vi "AlliGator Save FLI Dataset Metadata to HDF5.vi"(7 "Compression":bool, 8 "error in (no error)":errorcluster, 9 "Gate Names":string[](array[string])=["Gate"], 10 "Dataset Information":T1, 11 "Software + Version":string) -> (0 "error out":errorcluster, 2 "File Path out":path, 3 "HDF5 File ref out":T3 format="%.0x")   [LabVIEW 2021, in "AlliGator Files.lvlib"]
doc: "Saves the FLI Dataset metadata in the AlliGator HDF5 file format."
uses:
  AlliGator Files.lvlib
  <vilib>/addons/h5labview2/base/hid_t.ctl
  AlliGator Saved Dataset Information.ctl
  Phasor/Phasor Fluorescence Lifetime Parameters v3.ctl
  <vilib>/addons/h5labview2/file/H5Fmode.ctl
  AlliGator FLI Dataset HDF5 File Sections.ctl
  Source Image/AlliGator Image Binning Options.ctl
  <vilib>/addons/h5labview2/base/lib_path.vi
  <vilib>/addons/h5labview2/base/H5Equery.vi
  <vilib>/addons/h5labview2/dataset/H5Dwrite.llb/H5Dwrite.xnode
  <vilib>/addons/h5labview2/group/H5G.lvlib
  Strings/Strings.lvlib
  Utilities/Utilities.lvlib
  Source Image/AlliGator Source Image.lvlib
  <vilib>/addons/h5labview2/file/H5F.lvlib
  Phasor/Phasor.lvlib
panel:
  # "see the AlliGator License on the block diagram (Ctrl+E or Window:Show Block Diagram)"
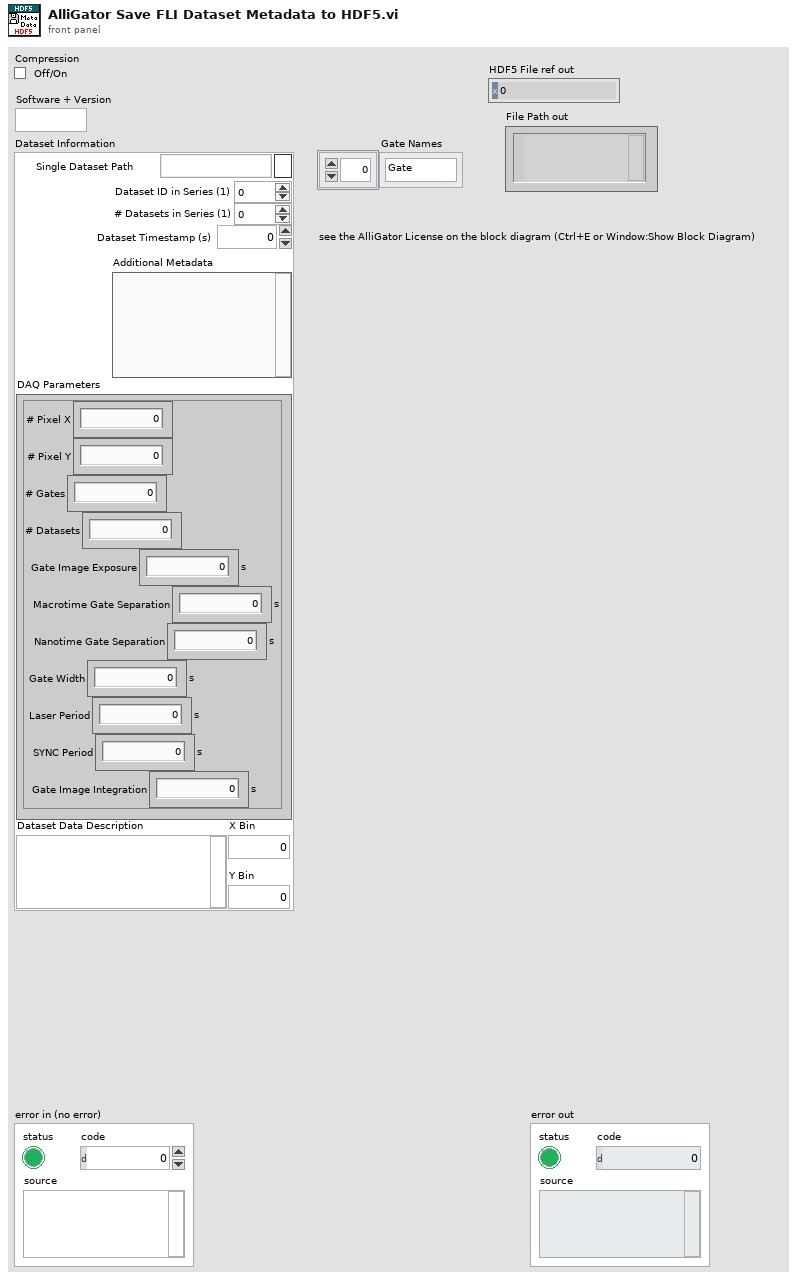
[diagram p1: front panel]
types:
  T1 = typedef "AlliGator Files.lvlib/AlliGator Saved Dataset Information.ctl" = cluster{"Single Dataset Path":path, "Dataset ID in Series (1)":i32, "# Datasets in Series (1)":i32, "Dataset Timestamp (s)":dbl, "Additional Metadata":string, "DAQ Parameters":T2, "Dataset Data Description":string, "X Bin":i32, "Y Bin":i32}
  T2 = typedef "Phasor.lvlib/Phasor Fluorescence Lifetime Parameters v3.ctl" = cluster{"# Pixel X":i32, "# Pixel Y":i32, "# Gates":i32, "# Datasets":i32, "Gate Image Exposure":dbl[unit], "Macrotime Gate Separation":dbl[unit], "Nanotime Gate Separation":dbl[unit], "Gate Width":dbl[unit], "Laser Period":dbl[unit], "SYNC Period":dbl[unit], "Gate Image Integration":dbl[unit]}
  T3 = typedef "hid_t.ctl" = i64
  T4 = typedef "AlliGator Files.lvlib/AlliGator FLI Dataset HDF5 File Sections.ctl" = enum16{"File Information", "DAQ Parameters", "Image Information", "Metadata"}
  T5 = typedef "H5F.lvlib/H5Fmode.ctl" = enum16{"read-only", "read-write", "overwrite", "create new", "open or create"}
  T6 = typedef "AlliGator Source Image.lvlib/AlliGator Image Binning Options.ctl" = cluster{"Use Image Binning":bool, "X Bin":i32, "Y Bin":i32}
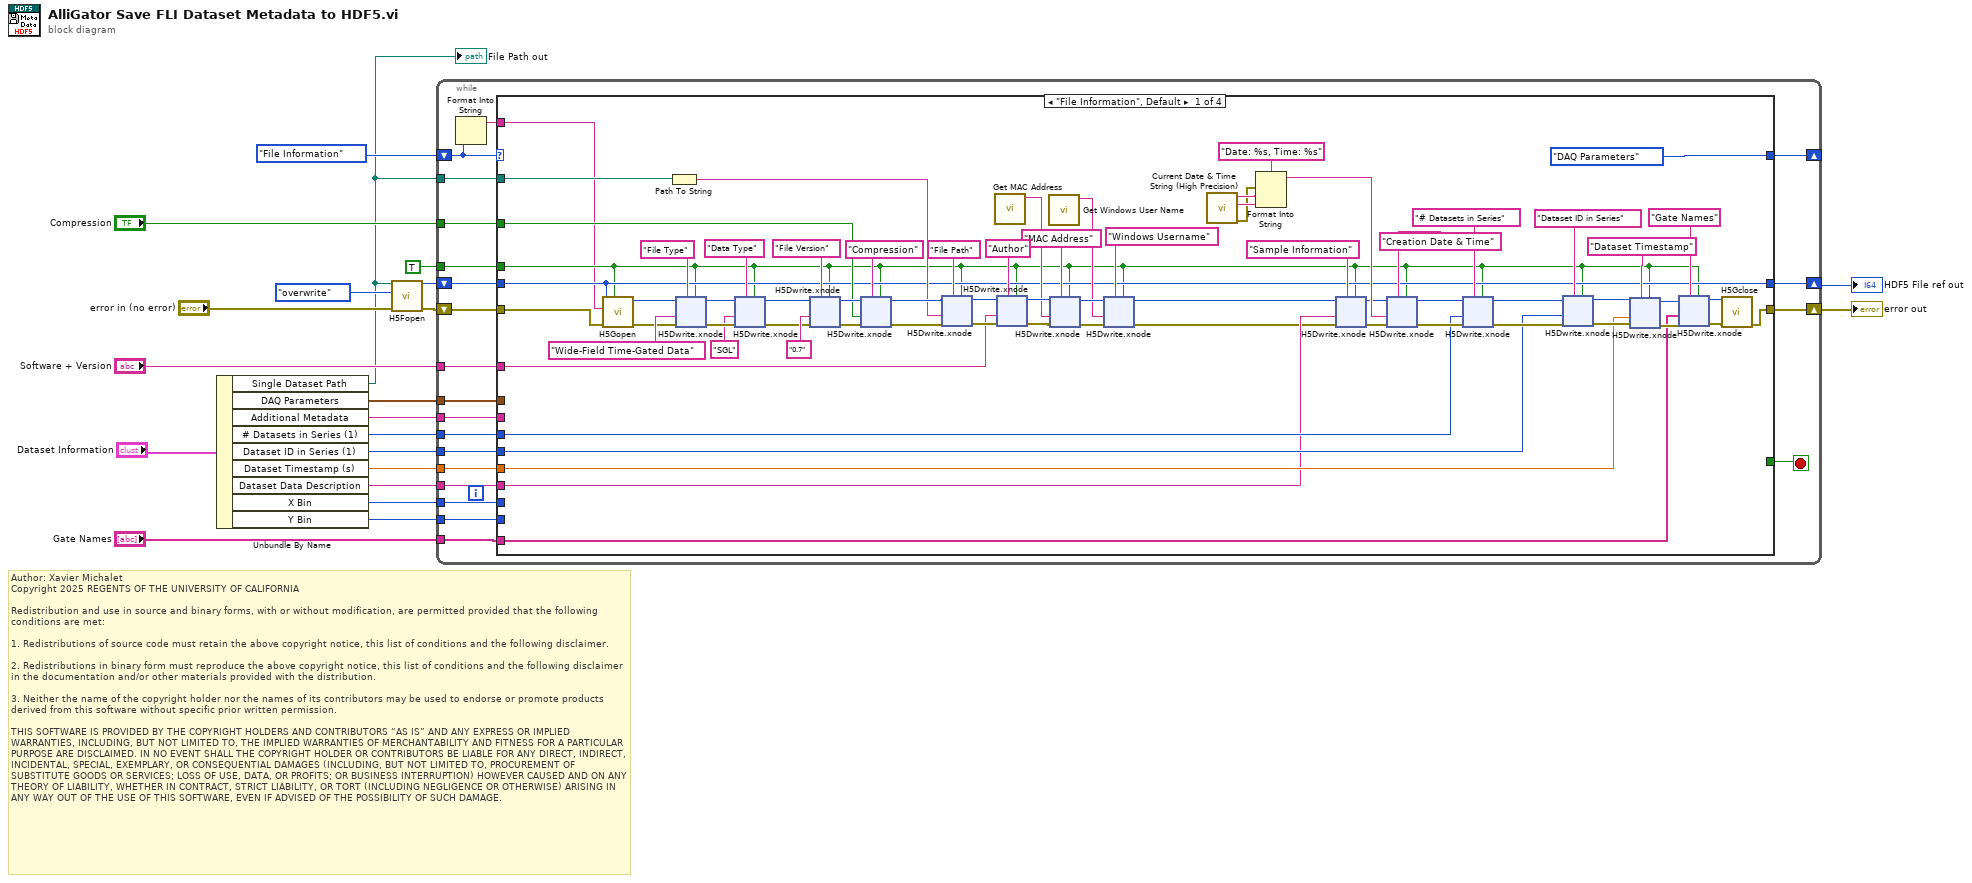
[diagram p0: block diagram]
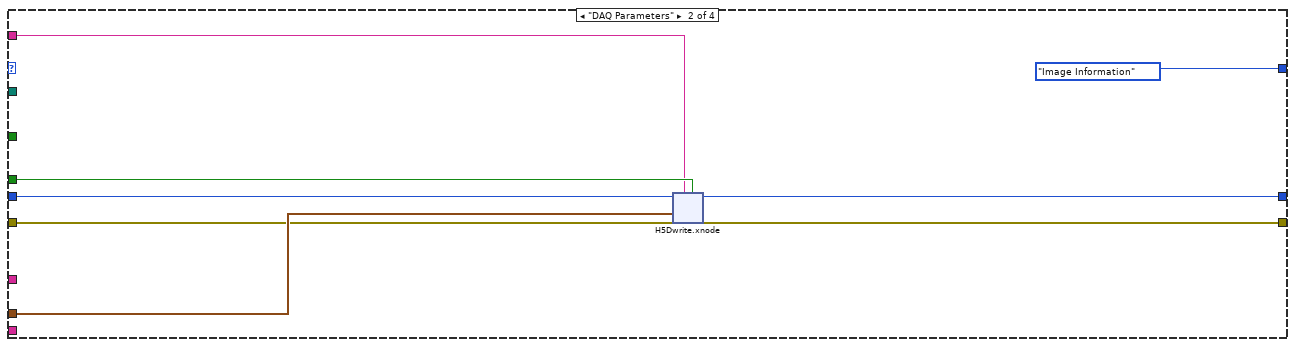
[diagram p2: hidden frame]
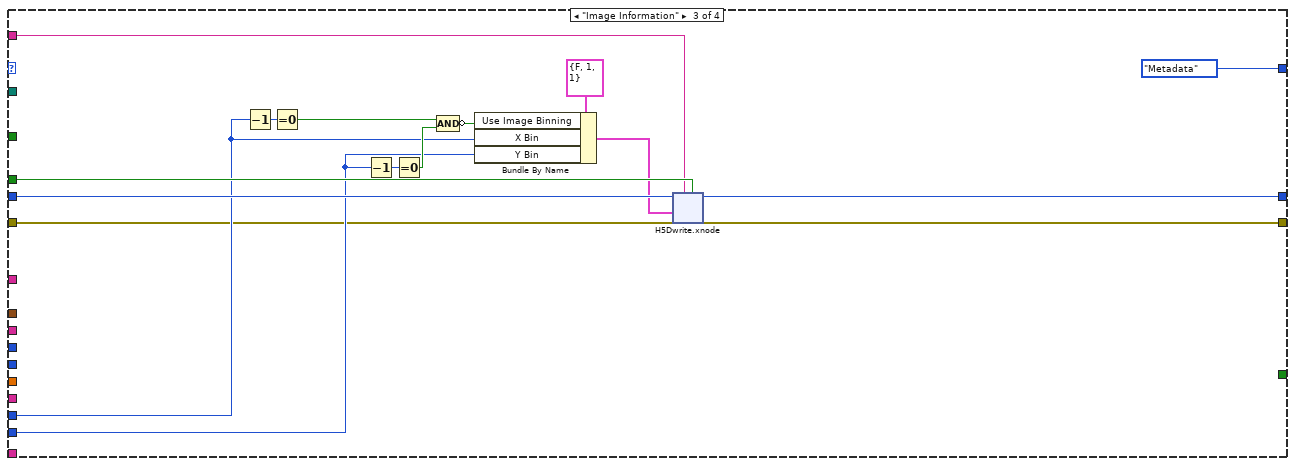
[diagram p3: hidden frame]
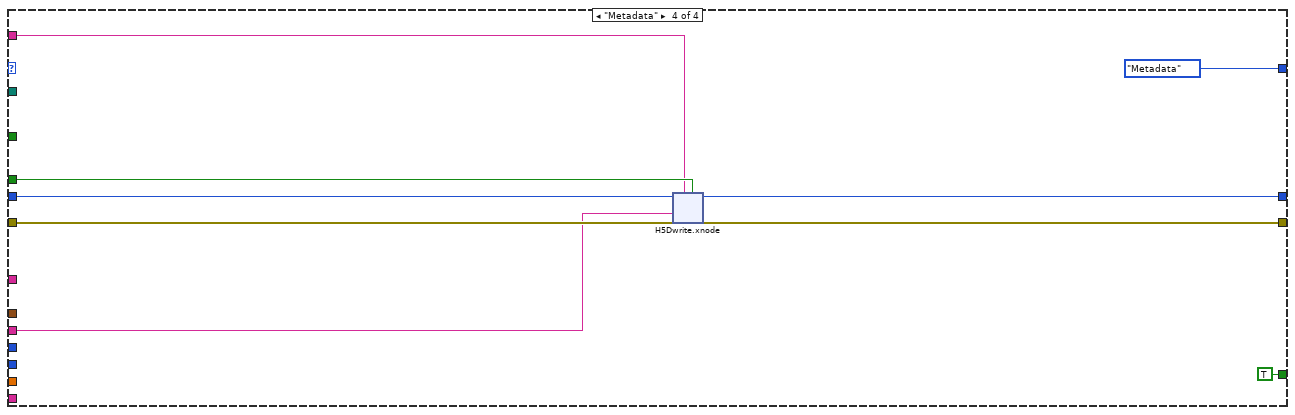
[diagram p4: hidden frame]
diagram:
  # "Author: Xavier Michalet\nCopyright 2025 REGENTS OF THE UNIVERSITY OF CALIFORNIA\n\nRedistribution and use in source and binary forms, with or without modification, are permitted provided that the following conditions are met:\n\n1. Redistributions of source code must retain the above copyright notice, this list of conditions and the following disclaimer.\n\n2. Redistributions in binary form must reproduce the above copyright notice, this list of conditions and the following disclaimer in the documentation and/or other materials provided with the distribution.\n\n3. Neither the name of the copyright holder nor the names of its contributors may be used to endorse or promote products derived from this software without specific prior written permission.\n\nTHIS SOFTWARE IS PROVIDED BY THE COPYRIGHT HOLDERS AND CONTRIBUTORS “AS IS” AND ANY EXPRESS OR IMPLIED WARRANTIES, INCLUDING, BUT NOT LIMITED TO, THE IMPLIED WARRANTIES OF MERCHANTABILITY AND FITNESS FOR A PARTICULAR PURPOSE ARE DISCLAIMED. IN NO EVENT SHALL THE COPYRIGHT HOLDER OR CONTRIBUTORS BE LIABLE FOR ANY DIRECT, INDIRECT, INCIDENTAL, SPECIAL, EXEMPLARY, OR CONSEQUENTIAL DAMAGES (INCLUDING, BUT NOT LIMITED TO, PROCUREMENT OF SUBSTITUTE GOODS OR SERVICES; LOSS OF USE, DATA, OR PROFITS; OR BUSINESS INTERRUPTION) HOWEVER CAUSED AND ON ANY THEORY OF LIABILITY, WHETHER IN CONTRACT, STRICT LIABILITY, OR TORT (INCLUDING NEGLIGENCE OR OTHERWISE) ARISING IN ANY WAY OUT OF THE USE OF THIS SOFTWARE, EVEN IF ADVISED OF THE POSSIBILITY OF SUCH DAMAGE."
  n1 = Unbundle By Name("Dataset Information") -> ("Single Dataset Path"=w1:path, "DAQ Parameters"=w13:T2, "Additional Metadata"=w15:string, "# Datasets in Series (1)"=w8:i32, "Dataset ID in Series (1)"=w9:i32, "Dataset Timestamp (s)"=w10:dbl, "Dataset Data Description"=w16:string, "X Bin"=w17:i32, "Y Bin"=w18:i32)
  "File Path out" <- w1
  n2 = call <vilib>:"H5Fopen.vi"("error in (no error)"="error in (no error)", "mode (read-only)"=H5Fmode."overwrite", "path"=w1) -> ("error out"=w3:errorcluster, "ref out"=w14:T3)  [unwired: 7 in]
  n3 = while {
    tunnel: "Compression" -> [w39]
    tunnel: "Software + Version" -> [w38]
    tunnel: w8 -> [w37]
    tunnel: w9 -> [w36]
    tunnel: w10 -> [w35]
    tunnel: w1 -> [w34]
    tunnel: "Gate Names" -> [w33]
    shift-right: [w40] -> w21
    shift-left: w3 -> [w42]
    tunnel: TRUE ("replace? (F)") -> [w32]
    shift-right: [w31] -> _
    shift-left: AlliGator_FLI_Dataset_HDF5_File_Sections."File Information" -> [w28]
    shift-right: [w30] -> w19
    shift-left: w14 -> [w41]
    tunnel: w13 -> [w29]
    tunnel: w15 -> [w26]
    tunnel: w16 -> [w24]
    tunnel: w17 -> [w23]
    tunnel: w18 -> [w22]
    stop <- w25 stop-if-true
    n4 = Format Into String(w28) -> (resulting string=w27:string)  [unwired: 3 in, 1 out]
    n5 = case shown="\"File Information\", Default" w28 {
      tunnel: w42 -> [w111 w383 w405 w447]
      tunnel: w41 -> [w48 w384 w420 w448]
      tunnel: [w104 w381 w418 w445] -> w40
      tunnel: w39 -> [w95 _ _ _]
      tunnel: w38 -> [w62 _ _ _]
      tunnel: w37 -> [w58 _ _ _]
      tunnel: w36 -> [w57 _ _ _]
      tunnel: w35 -> [w56 _ _ _]
      tunnel: w34 -> [w50 _ _ _]
      tunnel: w33 -> [w49 _ _ _]
      tunnel: w32 -> [w47 w380 w417 w444]
      tunnel: [AlliGator_FLI_Dataset_HDF5_File_Sections."DAQ Parameters" AlliGator_FLI_Dataset_HDF5_File_Sections."Image Information" AlliGator_FLI_Dataset_HDF5_File_Sections."Metadata" AlliGator_FLI_Dataset_HDF5_File_Sections."Metadata"] -> w31
      tunnel: [w48 w382 w419 w446] -> w30
      tunnel: w29 -> [_ w385 _ _]
      tunnel: w27 -> [w46 w379 w416 w443]
      tunnel: w26 -> [_ _ _ w442]
      tunnel: [_ _ _ TRUE] -> w25
      tunnel: w24 -> [w44 _ _ _]
      tunnel: w23 -> [_ _ w407 _]
      tunnel: w22 -> [_ _ w406 _]
      frame "File Information", Default {
        n6 = call <vilib>:"H5Gopen.vi"("create? (F)"=w47, "error in (no error)"=w111, "name"=w46, "ref in"=w48) -> ("error out"=w108:errorcluster, "group out"=w106:T3)  [unwired: 6 in]
        n7 = Path To String(path=w50) -> (string=w79:string)
        n8 = xnode "H5Dwrite.xnode"("replace? (F)"=w47, "dataset name"="File Type", "error in (no error)"=w108, "data"="Wide-Field Time-Gated Data" ("dataset name"), "ref in"=w106) -> ("error out"=w102:errorcluster, "ref out"=w103:T3)  [unwired: 2 in, 1 out]
        n9 = xnode "H5Dwrite.xnode"("replace? (F)"=w47, "dataset name"="Data Type", "error in (no error)"=w102, "data"="SGL" ("dataset name"), "ref in"=w103) -> ("error out"=w100:errorcluster, "ref out"=w101:T3)  [unwired: 2 in, 1 out]
        n10 = xnode "H5Dwrite.xnode"("replace? (F)"=w47, "dataset name"="File Version", "error in (no error)"=w100, "data"="0.7" ("dataset name"), "ref in"=w101) -> ("error out"=w96:errorcluster, "ref out"=w97:T3)  [unwired: 2 in, 1 out]
        n11 = xnode "H5Dwrite.xnode"("replace? (F)"=w47, "dataset name"="Compression", "error in (no error)"=w96, "data"=w95, "ref in"=w97) -> ("error out"=w82:errorcluster, "ref out"=w81:T3)  [unwired: 2 in, 1 out]
        n12 = xnode "H5Dwrite.xnode"("replace? (F)"=w47, "dataset name"="File Path", "error in (no error)"=w82, "data"=w79, "ref in"=w81) -> ("error out"=w92:errorcluster, "ref out"=w93:T3)  [unwired: 2 in, 1 out]
        n13 = call "Get MAC Address.vi"() -> ("MAC address"=w85:string)  [unwired: 10 in, 1 out]
        n14 = xnode "H5Dwrite.xnode"("replace? (F)"=w47, "dataset name"="Author", "error in (no error)"=w92, "data"=w62, "ref in"=w93) -> ("error out"=w90:errorcluster, "ref out"=w89:T3)  [unwired: 2 in, 1 out]
        n15 = call "Get Windows User Name.vi"() -> ("User Name"=w83:string)  [unwired: 10 in, 1 out]
        n16 = xnode "H5Dwrite.xnode"("replace? (F)"=w47, "dataset name"="MAC Address", "error in (no error)"=w90, "data"=w85, "ref in"=w89) -> ("error out"=w88:errorcluster, "ref out"=w87:T3)  [unwired: 2 in, 1 out]
        n17 = xnode "H5Dwrite.xnode"("replace? (F)"=w47, "dataset name"="Windows Username", "error in (no error)"=w88, "data"=w83, "ref in"=w87) -> ("error out"=w43:errorcluster, "ref out"=w71:T3)  [unwired: 2 in, 1 out]
        n18 = call "Current Date & Time String (High Precision).vi"() -> ("Error Out"=w76:errorcluster, "time string"=w77:string, "date string"=w78:string)  [unwired: 8 in, 1 out]
        n19 = Format Into String(format string="Date: %s, Time: %s", error in=w76, w78, w77) -> (resulting string=w73:string)  [unwired: 1 in, 1 out]
        n20 = xnode "H5Dwrite.xnode"("replace? (F)"=w47, "dataset name"="Sample Information" ("name"), "error in (no error)"=w43, "data"=w44, "ref in"=w71) -> ("error out"=w72:errorcluster, "ref out"=w70:T3)  [unwired: 2 in, 1 out]
        n21 = xnode "H5Dwrite.xnode"("replace? (F)"=w47, "dataset name"="Creation Date & Time", "error in (no error)"=w72, "data"=w73, "ref in"=w70) -> ("error out"=w65:errorcluster, "ref out"=w63:T3)  [unwired: 2 in, 1 out]
        n22 = xnode "H5Dwrite.xnode"("replace? (F)"=w47, "dataset name"="# Datasets in Series" ("name"), "error in (no error)"=w65, "data"=w58, "ref in"=w63) -> ("error out"=w64:errorcluster, "ref out"=w67:T3)  [unwired: 2 in, 1 out]
        n23 = xnode "H5Dwrite.xnode"("replace? (F)"=w47, "dataset name"="Dataset ID in Series" ("name"), "error in (no error)"=w64, "data"=w57, "ref in"=w67) -> ("error out"=w60:errorcluster, "ref out"=w61:T3)  [unwired: 2 in, 1 out]
        n24 = xnode "H5Dwrite.xnode"("replace? (F)"=w47, "dataset name"="Dataset Timestamp" ("name"), "error in (no error)"=w60, "data"=w56, "ref in"=w61) -> ("error out"=w55:errorcluster, "ref out"=w53:T3)  [unwired: 2 in, 1 out]
        n25 = xnode "H5Dwrite.xnode"("replace? (F)"=w47, "dataset name"="Gate Names", "error in (no error)"=w55, "data"=w49, "ref in"=w53) -> ("error out"=w54:errorcluster, "ref out"=w52:T3)  [unwired: 2 in, 1 out]
        n26 = call <vilib>:"H5Gclose.vi"("error in (no error)"=w54, "group in"=w52) -> ("error out"=w104:errorcluster)  [unwired: 9 in]
      }
      frame "DAQ Parameters" {
        n27 = xnode "H5Dwrite.xnode"("replace? (F)"=w380, "dataset name"=w379, "error in (no error)"=w383, "data"=w385, "ref in"=w384) -> ("error out"=w381:errorcluster, "ref out"=w382:T3)  [unwired: 2 in, 1 out]
      }
      frame "Image Information" {
        n28 = Decrement(x=w407) -> (x-1=w411:i32)
        n29 = Equal To 0?(x=w411) -> (x = 0?=w410:bool)
        n30 = Decrement(x=w406) -> (x-1=w412:i32)
        n31 = Equal To 0?(x=w412) -> (x = 0?=w409:bool)
        n32 = Compound Arithmetic op=AND(w410, w409) -> (invert w408:bool)
        n33 = Bundle By Name(cluster=T6 {"Use Image Binning"=FALSE, "X Bin"=1, "Y Bin"=1} ("Image Binning Options"), "Use Image Binning"=w408, "X Bin"=w407, "Y Bin"=w406) -> (w414:T6)
        n34 = xnode "H5Dwrite.xnode"("replace? (F)"=w417, "dataset name"=w416, "error in (no error)"=w405, "data"=w414, "ref in"=w420) -> ("error out"=w418:errorcluster, "ref out"=w419:i64)  [unwired: 2 in, 1 out]
      }
      frame "Metadata" {
        n35 = xnode "H5Dwrite.xnode"("replace? (F)"=w444, "dataset name"=w443, "error in (no error)"=w447, "data"=w442, "ref in"=w448) -> ("error out"=w445:errorcluster, "ref out"=w446:T3)  [unwired: 2 in, 1 out]
      }
    }
  }
  "error out" <- w21
  "HDF5 File ref out" <- w19
